vi "Calibrate NART DUT.vi"(0 "RFSA Device":refnum<k15>="VST1" caption="instrument handle", 3 "CART TCP Connection In":refnum<k5>, 5 "Measurement Handle In":T1, 7 "Frequency and Tx Gain":T4[](array[typedef]), 9 "Chain Mask List":u32[](array[numeric])=[1, 2] format="%x", 11 "error in (no error)":errorcluster, 12 "Path Loss, dB":dbl[][][](array[numeric]) format="%.2p", 13 "Measurement Timeout, sec":T2=10.0 format="%.3f") -> (4 "RFSA Handle Out":T3="RFSA" caption="RFSA Handle", 6 "Measurement Handle Out":T1, 8 "CART TCP Connection Out":refnum<k5>, 10 "Calibration Log":string, 15 "error out":errorcluster)   [LabVIEW 2012]
uses:
  TypeDef/TX Cal Data Rate.ctl
  <userlib>/niRF/niSystem/SA/Includes/niSYS - RFSA - INC - STYP - Handle.ctl
  <userlib>/niRF/niSystem/SA/Includes/niSYS - SA - INC - STYP - Timeout.ctl
  <userlib>/niRF/niBasic/SA/Waveform/Includes/niBASIC - SA - Waveform - INC - STYP - Measurement Handle.ctl
  <userlib>/niRF/niBasic/SA/Waveform/Includes/niBASIC - SA - Waveform - INC - STYP - State Element.ctl
  <userlib>/niRF/niSystem/SA/Includes/niSYS - SA - INC - STYP - Measurement Interval.ctl
  <userlib>/niRF/niSystem/SA/Includes/niSYS - SA - INC - STYP - RBW Filter.ctl
  <userlib>/niRF/niSystem/SA/Includes/niSYS - SA - INC - STYP - External Attenuation.ctl
  <userlib>/niRF/niBasic/SA/Waveform/Includes/niBASIC - SA - Waveform - INC - STYP - Averaging.ctl
  <userlib>/niRF/niSystem/SA/Includes/niSYS - SA - INC - STYP - Traces Active.ctl
  <userlib>/niRF/niSystem/SA/Includes/niSYS - SA - INC - STYP - Measurement Request.ctl
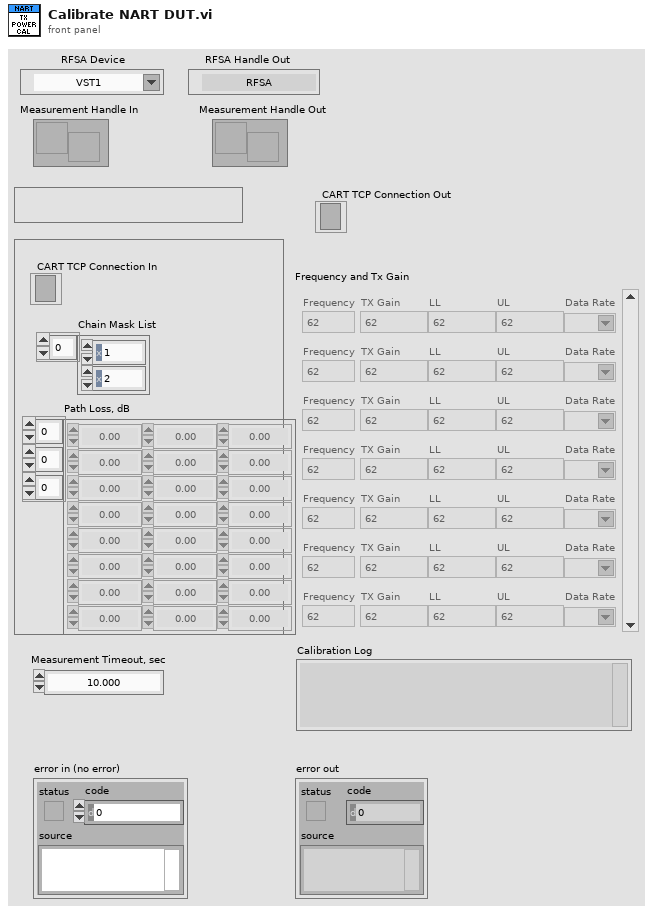
[diagram p1: front panel]
types:
  T1 = typedef "niBASIC - SA - Waveform - INC - STYP - Measurement Handle.ctl" = refnum<notifier>
  T2 = typedef "niSYS - SA - INC - STYP - Timeout.ctl" = dbl
  T3 = typedef "niSYS - RFSA - INC - STYP - Handle.ctl" = refnum<k15>
  T4 = typedef "TX Cal Data Rate.ctl" = cluster{"Frequency":u32, "TX Gain":u32, "LL":dbl, "UL":dbl, "Data Rate":string}
  T5 = typedef "niSYS - SA - INC - STYP - Measurement Interval.ctl" = dbl
  T6 = typedef "niSYS - SA - INC - STYP - Measurement Request.ctl" = enum16{"Measure", "Fetch", "Initiate"}
  T7 = cluster{"Frequency, MHz":u32, "TX Gain":u32, "Data Rate":string, "Packet Length":u32, "Packet Count":i32}
  T8 = typedef "niBASIC - SA - Waveform - INC - STYP - Measurement.ctl" = cluster{"Mean Power, dBm":dbl, "Peak to Average Ratio, dB":dbl, "Maximum Power, dBm":dbl, "Minimum Power, dBm":dbl}
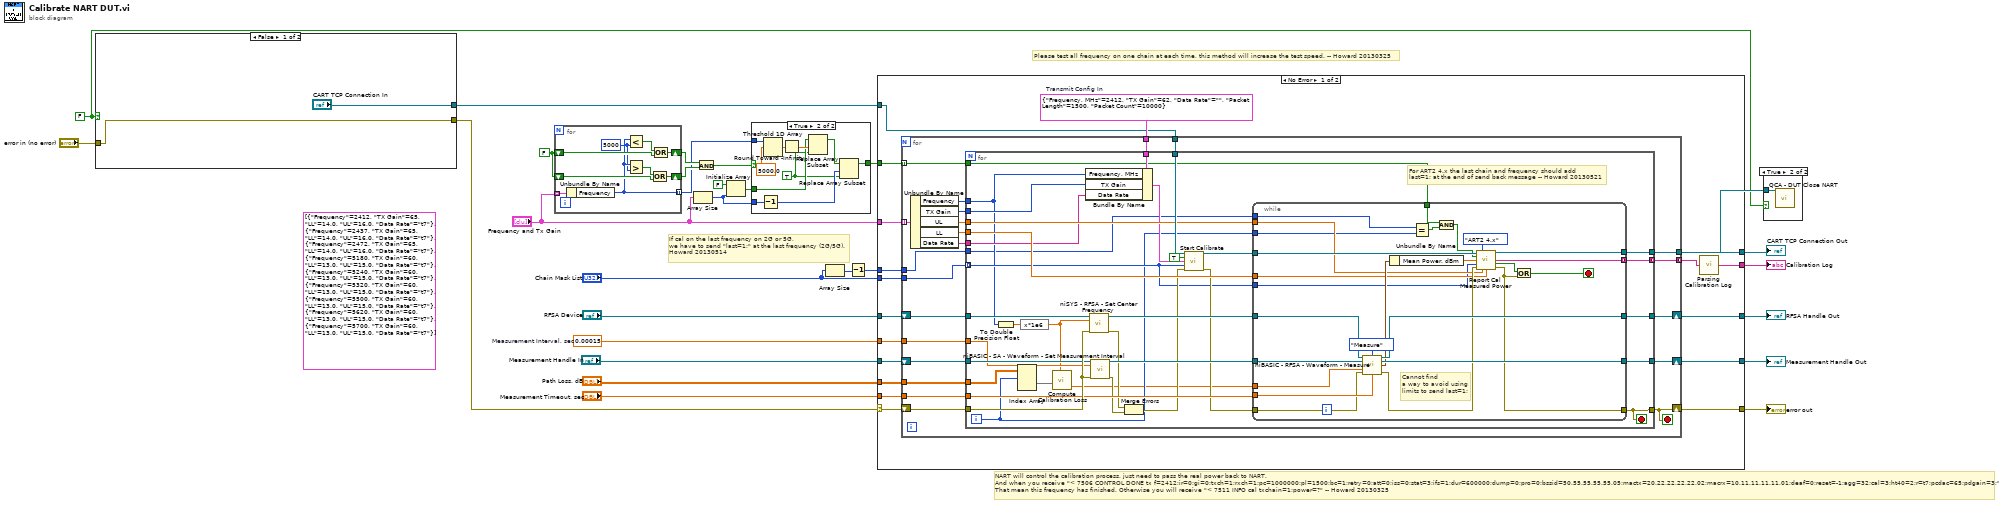
[diagram p0: block diagram]
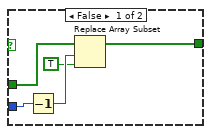
[diagram p2: hidden frame]
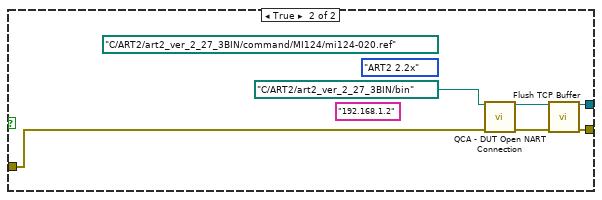
[diagram p4: hidden frame]
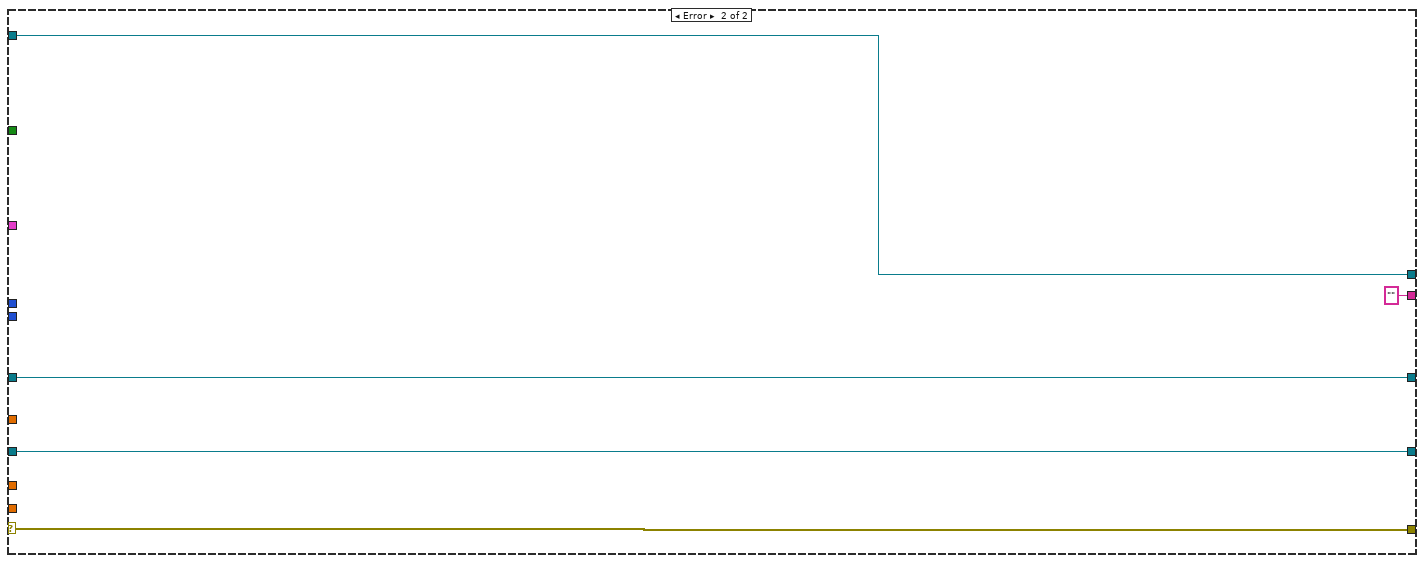
[diagram p5: hidden frame]
diagram:
  w16 = FALSE
  (unwired) T4[] [{"Frequency"=2412, "TX Gain"=65, "LL"=14.0, "UL"=16.0, "Data Rate"="t7"}, {"Frequency"=2437, "TX Gain"=65, "LL"=14.0, "UL"=16.0, "Data Rate"="t7"}, {"Frequency"=2472, "TX Gain"=65, "LL"=14.0, "UL"=16.0, "Data Rate"="t7"}, {"Frequency"=5180, "TX Gain"=60, "LL"=13.0, "UL"=15.0, "Data Rate"="t7"}, {"Frequency"=5240, "TX Gain"=60, "LL"=13.0, "UL"=15.0, "Data Rate"="t7"}, {"Frequency"=5320, "TX Gain"=60, "LL"=13.0, "UL"=15.0, "Data Rate"="t7"}, {"Frequency"=5500, "TX Gain"=60, "LL"=13.0, "UL"=15.0, "Data Rate"="t7"}, {"Frequency"=5620, "TX Gain"=60, "LL"=13.0, "UL"=15.0, "Data Rate"="t7"}, {"Frequency"=5700, "TX Gain"=60, "LL"=13.0, "UL"=15.0, "Data Rate"="t7"}] ("Frequency and Tx Gain")
  w18 = FALSE
  w23 = T5 0.00015  # Measurement Interval, sec
  # "If cal on the last frequency on 2G or 5G, \nwe have to send \"last=1;\" at the last frequency (2G/5G).\nHoward 20130514"
  # "Please test all frequency on one chain at each time, this method will increase the test speed. -- Howard 20130325"
  # "NART will control the calibration process, just need to pass the real power back to NART.\nAnd when you receive \"< 7506 CONTROL DONE tx f=2412;ir=0;gi=0;txch=1;rxch=1;pc=1000000;pl=1500;bc=1;retry=0;att=0;iss=0;stat=3;ifs=1;dur=600000;dump=0;pro=0;bssid=50.55.55.55.55.05;mactx=20.22.22.22.22.02;macrx=10.11.11.11.11.01;deaf=0;reset=-1;agg=32;cal=3;ht40=2;r=t7;pcdac=65;pdgain=3;\"\nThat mean this frequency has finished. Otherwise you will receive \"< 7511 INFO cal txchain=1;power=?\" -- Howard 20130325"
  n1 = case shown="False" w18 {
    tunnel: [w29 w33] -> w22
    tunnel: ["CART TCP Connection In" w32] -> w21
    tunnel: "error in (no error)" -> [w29 w31]
    frame False {
    }
    frame True {
      (unwired) path "C:/ART2/art2_ver_2_27_3BIN/command/MI124/mi124-020.ref" ("DUT Reference File For ART2 2.2x")
      (unwired) enum16{"ART2 2.2x", "ART2 4.x"}."ART2 2.2x" ("ART2 Version")
      (unwired) "192.168.1.2" ("IP Address (\"\": localhost)")
      n2 = call "QCA - DUT Open NART Connection.vi"("NART Directory"=path "C:/ART2/art2_ver_2_27_3BIN/bin", "error in (no error)"=w31) -> ("NART TCP Connection"=w35:refnum<k5>, "error out"=w34:errorcluster)  [unwired: 12 in]
      n3 = call "Flush TCP Buffer.vi"("CART TCP Connection In"=w35, "error in (no error)"=w34) -> ("CART TCP Connection Out"=w32:refnum<k5>, "error out"=w33:errorcluster)  [unwired: 12 in]
    }
  }
  n4 = for {
    tunnel: "Frequency and Tx Gain" -> [w44] mode=indexing
    tunnel: [w37] -> w7 mode=indexing
    shift-right: [w42] -> w14
    shift-left: w16 -> [w41]
    shift-right: [w43] -> w15
    shift-left: w16 -> [w40]
    w36 = u32 5000 ("y")
    n5 = Unbundle By Name(w44) -> ("Frequency"=w37:u32)
    n6 = Less?(x=w37, y=w36) -> (x < y?=w39:bool)
    n7 = Greater?(x=w37, y=w36) -> (0:w38:bool)
    n8 = Or(x=w38, y=w40) -> (x .or. y?=w43:bool)
    n9 = Or(x=w39, y=w41) -> (x .or. y?=w42:bool)
  }
  n10 = Array Size(array="Frequency and Tx Gain") -> (size(s)=w10:i32)
  n11 = And(x=w14, y=w15) -> (x .and. y?=w13:bool)
  n12 = Initialize Array(FALSE, w10) -> (w9:bool[])
  n13 = case shown="True" w13 {
    tunnel: w10 -> [w49 w56]
    tunnel: w9 -> [w47 w53]
    tunnel: [w45 w55] -> w8
    tunnel: w7 -> [_ w59]
    frame False {
      n14 = Decrement(x=w49) -> (x-1=w48:i32)
      n15 = Replace Array Subset(array=w47, new element=TRUE ("new element/subarray"), index=w48) -> (w45:bool[])
    }
    frame True {
      w50 = TRUE ("new element/subarray")
      n16 = Decrement(x=w56) -> (x-1=w51:i32)
      n17 = Threshold 1D Array(2:5000.0 ("threshold y"), 3:w59) -> (0:w57:dbl)  [unwired: 1 in]
      n18 = Round Toward -Infinity(1:w57) -> (0:w54:dbl)
      n19 = Replace Array Subset(array=w53, new element=w50, index=w54) -> (w52:bool[])
      n20 = Replace Array Subset(array=w52, new element=w50, index=w51) -> (w55:bool[])
    }
  }
  n21 = Array Size(array="Chain Mask List") -> (size(s)=w6:i32)
  n22 = Decrement(x=w6) -> (x-1=w4:i32)
  n23 = case shown="No Error" w22 {
    selector: w22 -> [w75 w165]
    tunnel: [w66 w165] -> w27
    tunnel: "Frequency and Tx Gain" -> [w76 _]
    tunnel: "Measurement Handle In" -> [w74 w163]
    tunnel: [w73 w163] -> w1
    tunnel: "RFSA Device" -> [w72 w164]
    tunnel: [w71 w164] -> w25
    tunnel: "Path Loss, dB" -> [w70 _]
    tunnel: "Measurement Timeout, sec" -> [w69 _]
    tunnel: w23 -> [w68 _]
    tunnel: w21 -> [w67 w162]
    tunnel: [w65 w162] -> w20
    tunnel: "Chain Mask List" -> [w64 _]
    tunnel: w8 -> [w63 _]
    tunnel: w4 -> [w62 _]
    tunnel: [w60 "" ("Calibration Log")] -> w3
    frame No Error {
      w77 = T7 {"Frequency, MHz"=2412, "TX Gain"=62, "Data Rate"="", "Packet Length"=1500, "Packet Count"=10000}  # Transmit Config In
      n24 = for {
        tunnel: w77 -> [w99]
        tunnel: w76 -> [w98] mode=indexing
        shift-right: [w97] -> w66
        shift-left: w75 -> [w96]
        shift-right: [w94] -> w73
        shift-left: w74 -> [w95]
        shift-right: [w92] -> w71
        shift-left: w72 -> [w93]
        tunnel: w70 -> [w91]
        tunnel: w69 -> [w90]
        tunnel: w68 -> [w89]
        tunnel: w67 -> [w88]
        tunnel: [w87] -> w65
        tunnel: w64 -> [w86]
        tunnel: w63 -> [w80] mode=indexing
        tunnel: w62 -> [w79]
        tunnel: [w78] -> w61 mode=concatenating
        stop <- w97 stop-if-true
        n25 = Unbundle By Name(w98) -> ("Frequency"=w85:u32, "TX Gain"=w82:u32, "UL"=w84:dbl, "LL"=w83:dbl, "Data Rate"=w81:string)
        n26 = for {
          tunnel: w99 -> [w134]
          tunnel: [w109] -> w97
          tunnel: w96 -> [w133]
          tunnel: w95 -> [w132]
          tunnel: [w131] -> w94
          tunnel: w93 -> [w130]
          tunnel: [w129] -> w92
          tunnel: w91 -> [w104]
          tunnel: w90 -> [w128]
          tunnel: w89 -> [w127]
          tunnel: w88 -> [w126]
          tunnel: [w125] -> w87
          tunnel: w86 -> [w108] mode=indexing
          tunnel: w85 -> [w107]
          tunnel: w84 -> [w124]
          tunnel: w83 -> [w123]
          tunnel: w82 -> [w122]
          tunnel: w81 -> [w121]
          tunnel: w80 -> [w106]
          tunnel: w79 -> [w105]
          tunnel: [w100] -> w78 mode=concatenating
          i -> [w103]
          stop <- w109 stop-if-true
          # "For ART2 4.x the last chain and frequency should add\nlast=1; at the end of send back message -- Howard 20130521"
          n27 = To Double Precision Float(number=w107) -> (double precision float=w116:dbl)
          n28 = Index Array(array=w104, index (dim 0)=w103) -> (element=w102:dbl[][])  [unwired: 2 in]
          n29 = expression code="x*1e6"(w116) -> (w111:dbl)
          n30 = call "Compute Calibration Loss.vi"("Table (frequency, power, pathloss)"=w102, "Center Frequency, Hz"=w111) -> ("External Attenuation, dB"=w101:dbl)  [unwired: 3 in, 2 out]
          n31 = Bundle By Name(cluster=w134, "Frequency, MHz"=w107, "TX Gain"=w122, "Data Rate"=w121) -> (w113:T7)
          n32 = call <userlib>:"niSYS - RFSA - Set Center Frequency.vi"("RFSA Handle In"=w130, "RFSA Center Frequency, Hz"=w111, "error in (no error)"=w133) -> ("RFSA Handle Out"=w119:T3, "error out"=w118:errorcluster)  [unwired: 11 out]
          n33 = call <userlib>:"niBASIC - SA - Waveform - Set Measurement Interval.vi"("Measurement Handle In"=w132, "Measurement Interval, sec"=w127, "error in (no error)"=w133) -> ("Measurement Handle Out"=w120:T1, "error out"=w117:errorcluster)  [unwired: 11 out]
          n34 = Merge Errors(w118, w117) -> (w114:errorcluster)
          n35 = call "Start Calibrate.vi"("CART TCP Connection In"=w126, "Send Cal Command?"=TRUE, "Calibrate Config"=w113, "Chain Mask"=w108, "error in (no error)"=w114) -> ("CART TCP Connection Out"=w112:refnum<k5>, "error out"=w115:errorcluster)  [unwired: 6 in, 3 out]
          n36 = while {
            tunnel: w120 -> [w160]
            tunnel: [w159] -> w131
            tunnel: [w158] -> w129
            tunnel: w128 -> [w157]
            tunnel: w119 -> [w156]
            tunnel: [w136] -> w109
            tunnel: w115 -> [w155]
            tunnel: w112 -> [w154]
            tunnel: [w153] -> w125
            tunnel: w101 -> [w145]
            tunnel: w123 -> [w147]
            tunnel: w124 -> [w148]
            tunnel: w108 -> [w146]
            tunnel: w106 -> [w143]
            tunnel: w103 -> [w142]
            tunnel: w105 -> [w141]
            tunnel: [w138] -> w100 mode=concatenating
            stop <- w135 stop-if-true
            # "Cannot find\na way to avoid using\nlimits to send last=1;"
            n37 = call <userlib>:"niBASIC - RFSA - Waveform - Measure.vi"("RFSA Handle In"=w156, "Measurement Request"=niSYS_-_SA_-_INC_-_STYP_-_Measurement_Request."Measure", "Measurement Handle In"=w160, "External Attenuation, dB"=w145, "error in (no error)"=w155, "Timeout, sec"=w157) -> ("RFSA Handle Out"=w158:T3, "Measurement Handle Out"=w159:T1, "Measurement"=w151:T8, "error out"=w150:errorcluster)  [unwired: 2 in, 4 out]
            n38 = Unbundle By Name(w151) -> ("Mean Power, dBm"=w144:dbl)
            n39 = Equal?(x=w141, y=w142) -> (x = y?=w140:bool)
            n40 = And(x=w143, y=w140) -> (x .and. y?=w139:bool)
            n41 = call "Report Cal Measured Power.vi"("CART TCP Connection In"=w154, "ART2 Version"=enum16{"ART2 2.2x", "ART2 4.x"}."ART2 4.x", "Commit?"=w139, "Measured Cal Power"=w144, "Chain Mask"=w146, "error in (no error)"=w150, "UL"=w148, "LL"=w147) -> ("CART TCP Connection Out"=w153:refnum<k5>, "Message Log"=w138:string[], "Done?"=w137:bool, "error out"=w136:errorcluster)  [unwired: 4 in]
            n42 = Or(x=w137, y=w136) -> (x .or. y?=w135:bool)
          }
        }
      }
      n43 = call "Parsing Calibration Log.vi"("Message Log"=w61) -> ("Calibration Log"=w60:string)
    }
    frame Error {
    }
  }
  "error out" <- w27
  "RFSA Handle Out" <- w25
  "CART TCP Connection Out" <- w20
  "Calibration Log" <- w3
  "Measurement Handle Out" <- w1
  n44 = case shown="True" w18 {
    tunnel: w20 -> [_ w166]
    frame False {
    }
    frame True {
      n45 = call "QCA - DUT Close NART.vi"("CART TCP Connection"=w166) -> ()  [unwired: 14 in, 1 out]
    }
  }
